vi "Configure Front Panel View.vi"(8 "error in":errorcluster, 10 "Show All":bool, 11 "DeepU Test Stand in":refnum<class "DeepU Test Stand.lvclass">) -> (0 "error out":errorcluster, 3 "DeepU Test Stand out":refnum<class "DeepU Test Stand.lvclass">)   [LabVIEW 2019, in "Test Stands.lvlib" / "DeepU Test Stand.lvclass"]
uses:
  DeepU Test Stand.lvclass
  C:/Users/wg/Documents/LV_Projects/test-stand/App/Generic Test Stand/Generic Test Stand.lvclass
  Generic Test Stand/TS Panel Method.ctl
  Generic Test Stand/Generic Test Stand.lvclass/Generic Test Stand.ctl
  DeepU Test Stand.lvclass/DeepU Test Stand.ctl
  DAC/DAC.lvclass
  Generic Test Stand/Generic Test Stand.lvclass
  Results/DeepU Results/DeepU Results.lvclass
  Results/Results Method.ctl
  Results/Results.lvlib
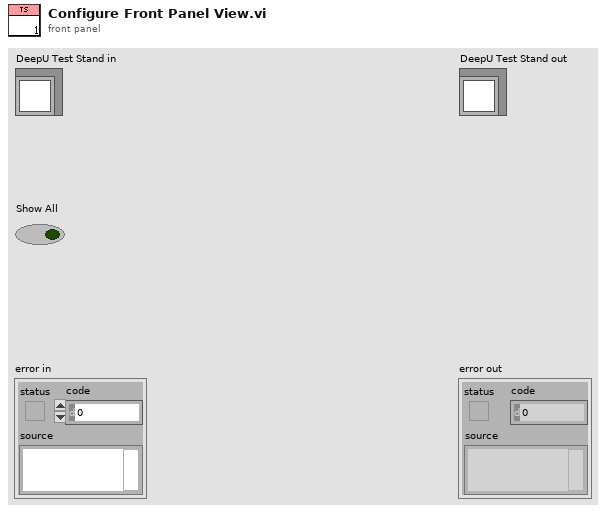
[diagram p1: front panel]
types:
  T1 = typedef "Generic Test Stand.lvclass/TS Panel Method.ctl" = enum16{"Send to Panel", "Receive from Panel", "Update Panel View"}
  T2 = typedef "Results.lvlib/Results Method.ctl" = enum16{"Get", "Set"}
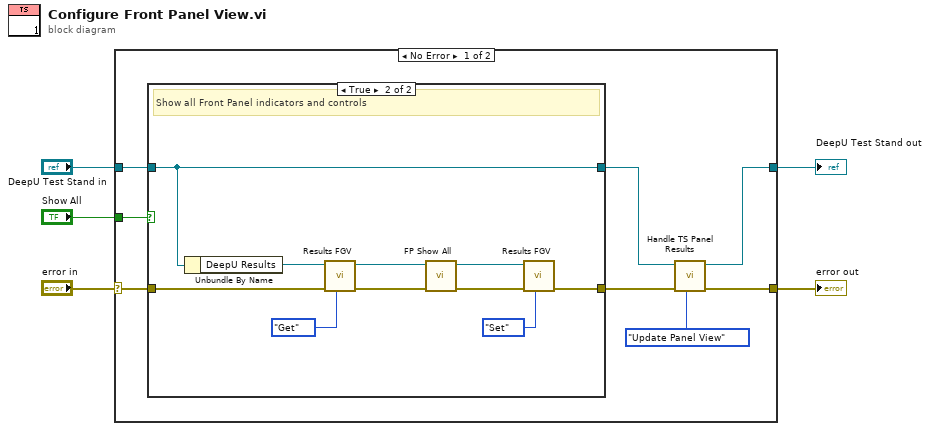
[diagram p0: block diagram]
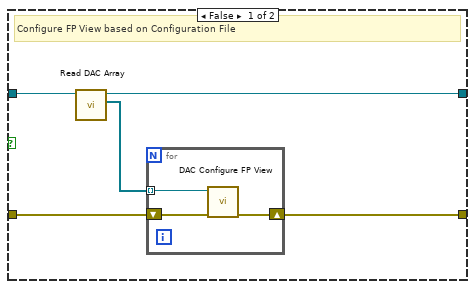
[diagram p2: hidden frame]
diagram:
  n1 = case shown="No Error" "error in" {
    selector: "error in" -> [w12 w33]
    tunnel: [w9 w33] -> w2
    tunnel: [w7 w32] -> w4
    tunnel: "DeepU Test Stand in" -> [w13 w32]
    tunnel: "Show All" -> [w6 _]
    frame No Error {
      n2 = case shown="True" w6 {
        tunnel: w13 -> [w18 w31]
        tunnel: w12 -> [w16 w27]
        tunnel: [w15 w24] -> w11
        tunnel: [w14 w31] -> w8
        frame False {
          # "Configure FP View based on Configuration File"
          n3 = call "Read DAC Array.vi"("Generic Test Stand in"=w18) -> ("DAC Array"=w17:refnum<class "DAC.lvclass">[], "Generic Test Stand out"=w14:refnum<class "DeepU Test Stand.lvclass">)  [unwired: 8 in, 1 out]
          n4 = for {
            tunnel: w17 -> [w21] mode=indexing
            shift-right: [w19] -> w15
            shift-left: w16 -> [w20]
            n5 = call-dynamic "DAC Configure FP View.vi"("error in"=w20, "DAC in"=w21) -> ("error out"=w19:errorcluster)  [unwired: 8 in, 1 out]
          }
        }
        frame True {
          # "Show all Front Panel indicators and controls"
          n6 = Unbundle By Name(w31) -> ("DeepU Results"=w30:refnum<class "DeepU Results.lvclass">)
          n7 = call-dynamic "Results FGV.vi"("Method"=Results_Method."Get", "error in"=w27, "DeepU Results in"=w30) -> ("error out"=w26:errorcluster, "DeepU Results out"=w23:refnum<class "DeepU Results.lvclass">)  [unwired: 7 in]
          n8 = call "FP Show All.vi"("error in (no error)"=w26, "DeepU Results in"=w23) -> ("error out"=w25:errorcluster, "DeepU Results out"=w22:refnum<class "DeepU Results.lvclass">)  [unwired: 8 in]
          n9 = call-dynamic "Results FGV.vi"("Method"=Results_Method."Set", "error in"=w25, "DeepU Results in"=w22) -> ("error out"=w24:errorcluster)  [unwired: 7 in, 1 out]
        }
      }
      n10 = call-dynamic "Handle TS Panel Results.vi"("Method"=TS_Panel_Method."Update Panel View", "error in"=w11, "DeepU Test Stand in"=w8) -> ("error out"=w9:errorcluster, "DeepU Test Stand out"=w7:refnum<class "DeepU Test Stand.lvclass">)  [unwired: 7 in]
    }
    frame Error {
    }
  }
  "error out" <- w2
  "DeepU Test Stand out" <- w4
